vi "Intermittency.vi"(2 "Block No":i32=1, 3 "Index":i32, 4 "Calib Constants":dbl[](array[numeric]) format="%.2f", 5 "C":dbl[](array[numeric]) format="%.2f", 6 "Shift in Before Fast Response":dbl[](array[numeric]) format="%.2f", 7 "Shift in After Fast Response":dbl[](array[numeric]) format="%.2f") -> (0 "Results":string[](array[string]), 1 "Shift Out":dbl[](array[numeric]) format="%.2f")   [LabVIEW 2010]
uses:
  Globals/Meas_global.vi
panel:
  # "Intermittency\nBkgnd Value\nThreshold"
  # "A                 B                   C                 Bkgnd     Bkgnd variance"
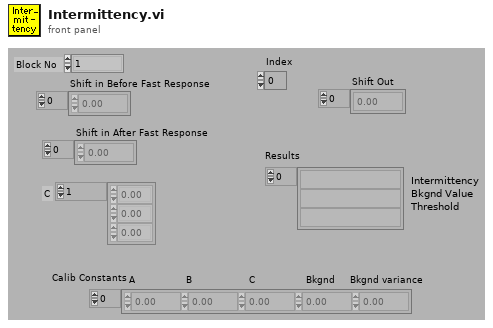
[diagram p1: front panel]
types:
  T1 = typedef "Analysis_info_cluster.ctl" = cluster{"Colour":u32, "Inst type":T2, "Inst name":string, "Symbol":string, "Code name":string, "Extra Info":string, "Inst Array":T3, "Index":i32, "Voltage Index":i32, "Extra Titles":string[], "Extra Values":string[]}
  T2 = typedef "Inst_type.ctl" = enum16{"Propeller anemometer", "Raw voltage", "Pressure Transducer", "Pitot-static tube", "Preston tube", "Hot wire", "Cross wire 1", "Cross wire 2", "Generic Linear", "Generic Polynomial", "Generic BackPoly", "Fast FID", "Thermocouple", "Cold wire", "Pulsed Wire", "LDA Vel", "LDA Tran time", "LDA Arr time"}
  T3 = typedef "Instrument_Array.ctl" = enum16{"PWA", "LDA", "Analogue"}
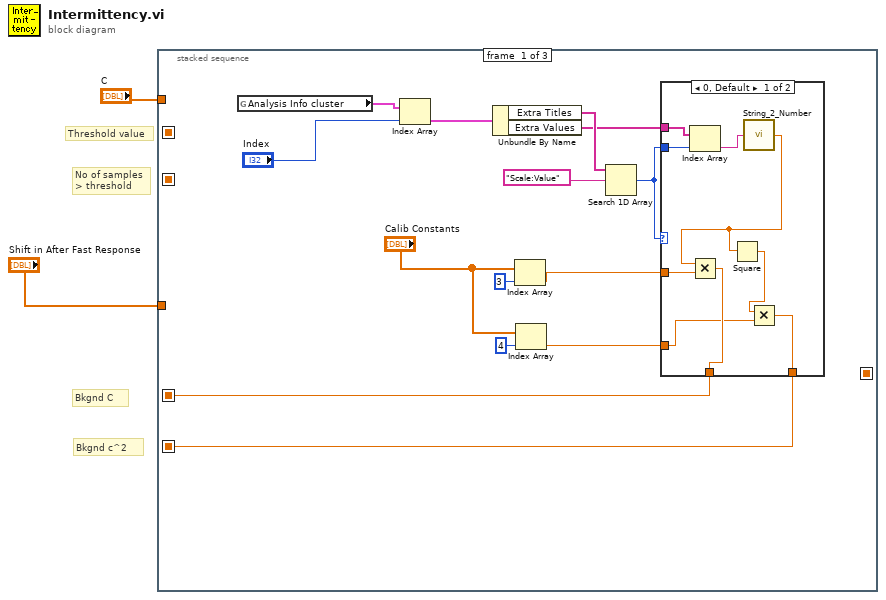
[diagram p0: block diagram]
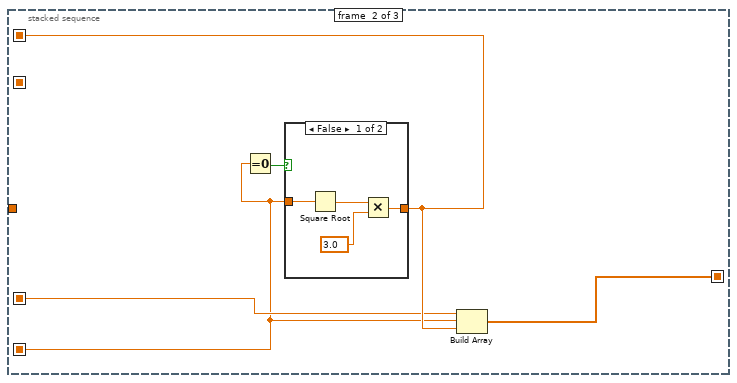
[diagram p3: hidden frame]
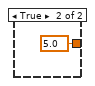
[diagram p4: hidden frame]
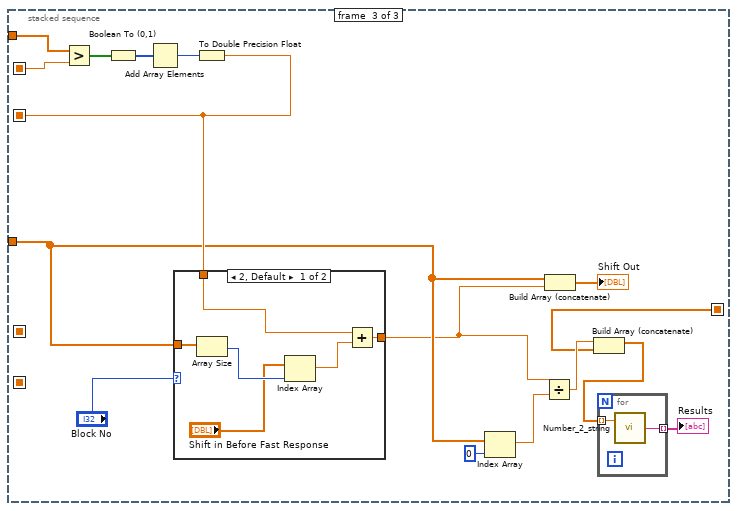
[diagram p5: hidden frame]
diagram:
  # "Bkgnd C"
  # "Bkgnd c^2"
  # "No of samples\n> threshold"
  # "Threshold value"
  n1 = stacked-sequence {
    seq-local: [_ w30 _] -> [_ _ w53]
    seq-local: [_ _ w47] -> [_ _ _]
    seq-local: [_ w32 _] -> [_ _ w40]
    seq-local: [w8 _ _] -> [_ w29 _]
    seq-local: [w6 _ _] -> [_ w28 _]
    tunnel: "C" -> [_ _ w52]
    tunnel: "Shift in After Fast Response" -> [_ _ w44]
    frame #0 {
      n2 = global read "Meas_global.vi" "Analysis Info cluster"() -> (w16:T1[])
      n3 = Index Array(array=w16, index="Index") -> (element=w14:T1)
      n4 = Unbundle By Name(w14) -> ("Extra Titles"=w13:string[], "Extra Values"=w3:string[])
      n5 = Index Array(array="Calib Constants", index=3 ("Index")) -> (element=w7:dbl)
      n6 = Index Array(array="Calib Constants", index=4 ("Index")) -> (element=w5:dbl)
      n7 = Search 1D Array(1D array=w13, element="Scale:Value") -> (index of element=w4:i32)  [unwired: 1 out]
      n8 = case shown="0, Default" w4 {
        tunnel: [w21 w27] -> w8
        tunnel: w7 -> [w22 w27]
        tunnel: [w17 w26] -> w6
        tunnel: w5 -> [w19 w26]
        tunnel: w4 -> [w25 _]
        tunnel: w3 -> [w24 _]
        frame 0, Default {
          n9 = Index Array(array=w24, index=w25) -> (element=w23:string)
          n10 = call "String_2_Number.vi"("Value"=w23) -> ("Numeric"=w20:dbl)
          n11 = Multiply(x=w20, y=w22) -> (x*y=w21:dbl)
          n12 = Square(x=w20) -> (x^2=w18:dbl)
          n13 = Multiply(x=w18, y=w19) -> (x*y=w17:dbl)
        }
        frame -1 {
        }
      }
    }
    frame #1 {
      n14 = Equal To 0?(x=w28) -> (x = 0?=w31:bool)
      n15 = case shown="False" w31 {
        tunnel: [w34 5.0] -> w30
        tunnel: w28 -> [w33 _]
        frame False {
          n16 = Square Root(x=w33) -> (sqrt(x)=w36:dbl)
          n17 = Multiply(x=w36, y=3.0) -> (x*y=w34:dbl)
        }
        frame True {
        }
      }
      n18 = Build Array(w29, w28, w30) -> (w32:dbl[])
    }
    frame #2 {
      n19 = Greater?(x=w52, y=w53) -> (0:w51:bool[])
      n20 = Boolean To (0,1)(Boolean=w51) -> (0, 1=w50:i16[])
      n21 = Add Array Elements(numeric array=w50) -> (sum=w48:i16)
      n22 = To Double Precision Float(number=w48) -> (double precision float=w47:dbl)
      n23 = case shown="2, Default" "Block No" {
        tunnel: w47 -> [w57 w62]
        tunnel: w44 -> [w61 _]
        tunnel: [w56 w62] -> w42
        frame 2, Default {
          n24 = Array Size(array=w61) -> (size(s)=w60:i32)
          n25 = Index Array(array="Shift in Before Fast Response", index=w60) -> (element=w58:dbl)
          n26 = Add(x=w57, y=w58) -> (x+y=w56:dbl)
        }
        frame 1 {
        }
      }
      n27 = Index Array(array=w44, index=0 ("Index")) -> (element=w43:dbl)
      n28 = Divide(x=w42, y=w43) -> (x/y=w41:dbl)
      n29 = Build Array (concatenate)(w44, w42) -> (→"Shift Out":dbl[])
      n30 = Build Array (concatenate)(w41, w40) -> (w39:dbl[])
      n31 = for {
        tunnel: w39 -> [w55] mode=indexing
        tunnel: [w54] -> w38 mode=indexing
        n32 = call "Number_2_string.vi"("number"=w55) -> ("String"=w54:string)  [unwired: 1 in]
      }
      "Results" <- w38
    }
  }
